vi "in_1d interp.vi"(7 "method":i32(ring) items=["nearest", "linear", "spline", "cubic Hermite", "Lagrange"], 9 "xi":dbl[](array[numeric]), 10 "Y":dbl[](array[numeric]), 11 "X":dbl[](array[numeric])) -> (0 "error":i32, 3 "yi":dbl[](array[numeric]))   [LabVIEW 2020, in "NI_Gmath.lvlib"]
uses:
  NI_Gmath.lvlib
  Scalar Polynomial Evaluation (DBL).vi
  NI_AALPro.lvlib
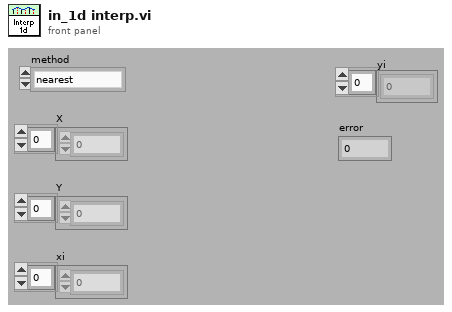
[diagram p1: front panel]
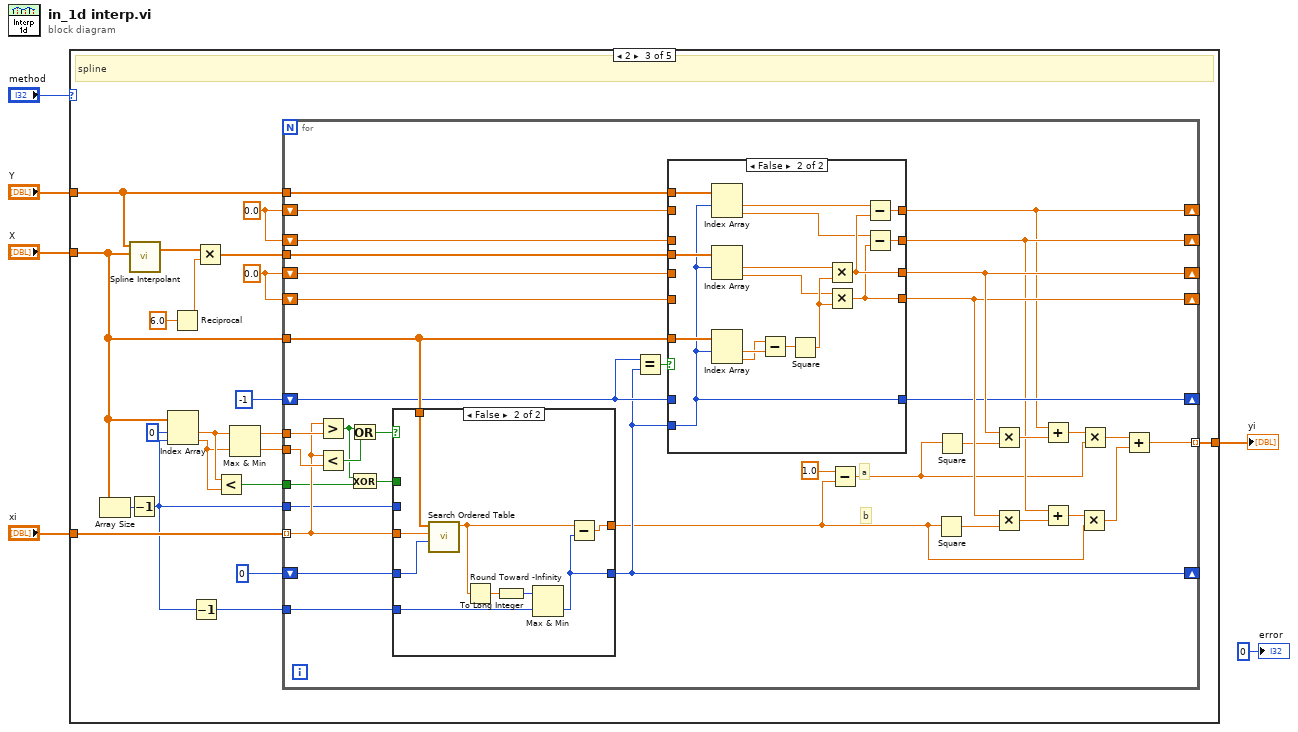
[diagram p0: block diagram]
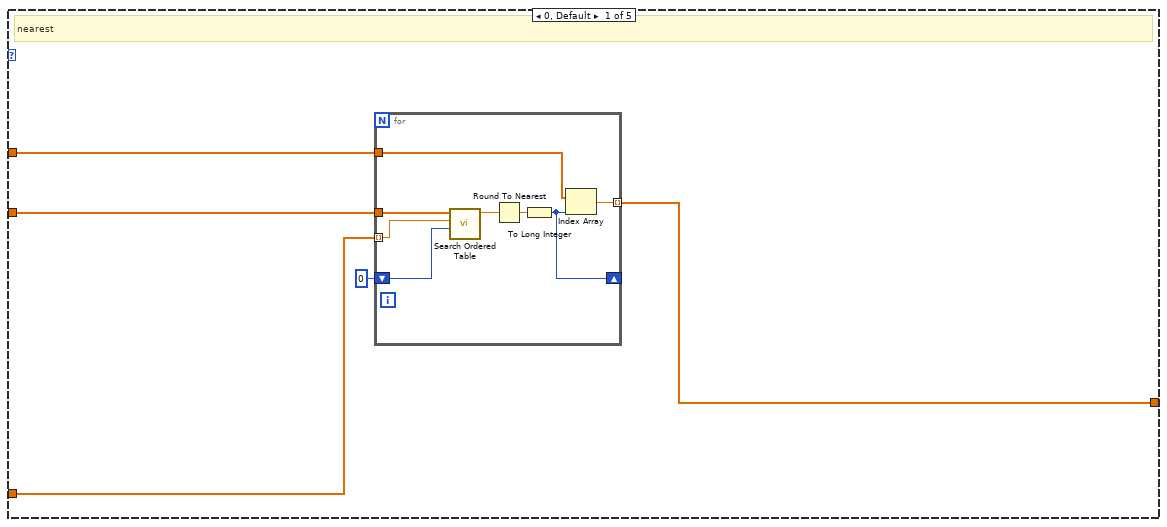
[diagram p2: hidden frame]
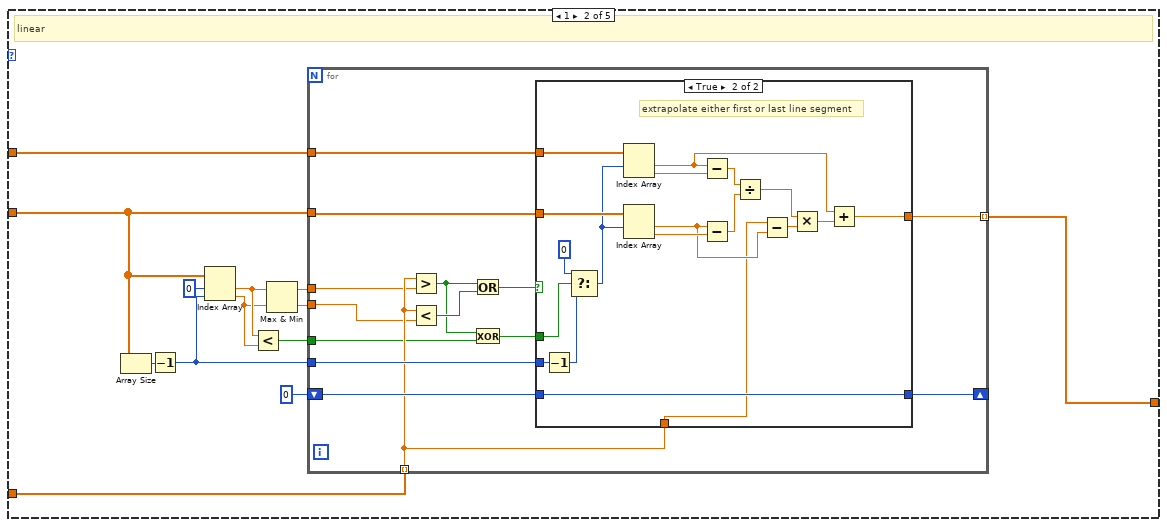
[diagram p3: hidden frame]
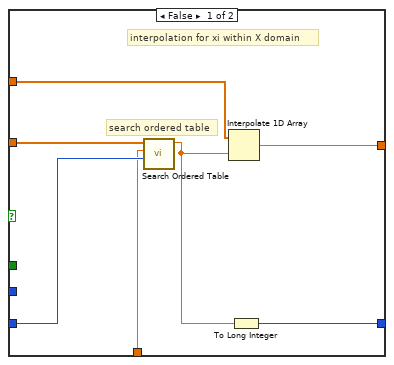
[diagram p4: hidden frame]
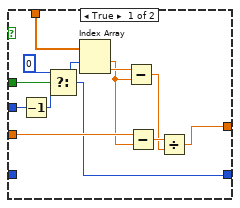
[diagram p5: hidden frame]
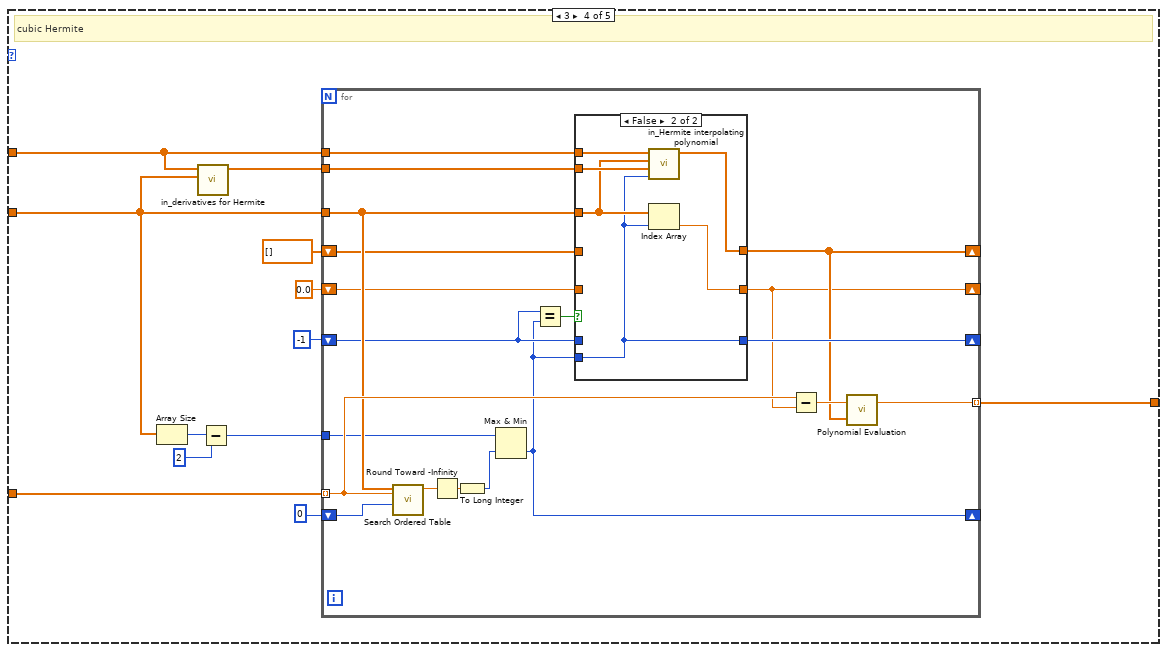
[diagram p7: hidden frame]
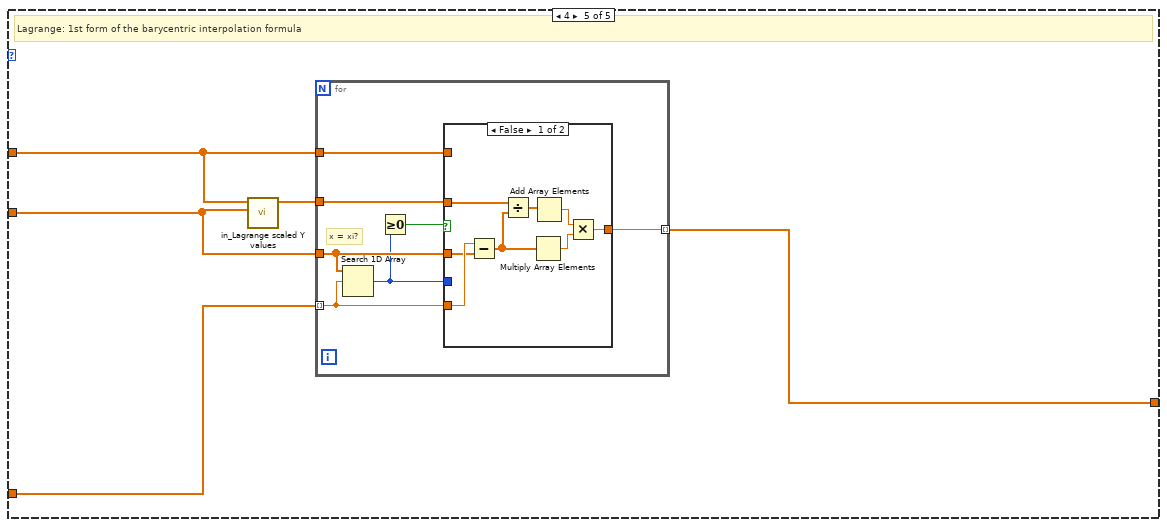
[diagram p9: hidden frame]
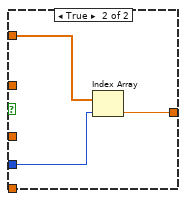
[diagram p10: hidden frame]
diagram:
  n1 = case shown="2" "method" {
    tunnel: "Y" -> [w7 w32 w93 w182 w214]
    tunnel: "X" -> [w9 w29 w78 w175 w217]
    tunnel: "xi" -> [w11 w26 w90 w185 w218]
    tunnel: [w10 w25 w92 w183 w215] -> w3
    frame 0, Default {
      # "nearest"
      n2 = for {
        tunnel: w9 -> [w16]
        tunnel: w11 -> [w15] mode=indexing
        tunnel: w7 -> [w18]
        tunnel: [w17] -> w10 mode=indexing
        shift-right: [w12] -> _
        shift-left: 0 -> [w14]
        n3 = call "Search Ordered Table.vi"("starting index"=w14, "x value"=w15, "ordered x array"=w16) -> ("fractional index"=w13:dbl)  [unwired: 8 in]
        n4 = Round To Nearest(number=w13) -> (nearest integer value=w19:dbl)
        n5 = To Long Integer(number=w19) -> (32bit integer=w12:i32)
        n6 = Index Array(array=w18, index=w12) -> (element=w17:dbl)
      }
    }
    frame 1 {
      # "linear"
      n7 = Array Size(array=w29) -> (size(s)=w30:i32)
      n8 = Decrement(x=w30) -> (x-1=w28:i32)
      n9 = Index Array(array=w29, index #1=0 ("index"), index #2=w28) -> (element #1=w23:dbl, element #2=w22:dbl)
      n10 = Less?(x=w23, y=w22) -> (x < y?=w24:bool)
      n11 = Max & Min(x=w23, y=w22) -> (max(x,y)=w21:dbl, min(x,y)=w20:dbl)
      n12 = for {
        tunnel: w29 -> [w46]
        tunnel: w32 -> [w45]
        tunnel: [w44] -> w25 mode=indexing
        tunnel: w20 -> [w33]
        tunnel: w21 -> [w34]
        tunnel: w28 -> [w42]
        shift-right: [w40] -> _
        shift-left: 0 ("index") -> [w41]
        tunnel: w26 -> [w39] mode=indexing
        tunnel: w24 -> [w38]
        n13 = Greater?(x=w39, y=w34) -> (0:w35:bool)
        n14 = Less?(x=w39, y=w33) -> (x < y?=w37:bool)
        n15 = Or(x=w35, y=w37) -> (x .or. y?=w43:bool)
        n16 = Exclusive Or(1:w38, 2:w35) -> (0:w36:bool)
        n17 = case shown="True" w43 {
          tunnel: w46 -> [w51 w72]
          tunnel: w45 -> [w53 w71]
          tunnel: [w52 w70] -> w44
          tunnel: w36 -> [_ w58]
          tunnel: w42 -> [_ w69]
          tunnel: w41 -> [w50 w55]
          tunnel: [w47 w55] -> w40
          tunnel: w39 -> [w49 w54]
          frame False {
            # "search ordered table"
            # "interpolation for xi within X domain"
            n18 = call "Search Ordered Table.vi"("starting index"=w50, "x value"=w49, "ordered x array"=w51) -> ("fractional index"=w48:dbl)  [unwired: 8 in]
            n19 = Interpolate 1D Array(1:w48, 2:w53) -> (0:w52:dbl)
            n20 = To Long Integer(number=w48) -> (32bit integer=w47:i32)
          }
          frame True {
            # "extrapolate either first or last line segment"
            n21 = Decrement(x=w69) -> (x-1=w59:i32)
            n22 = Select(t=0, s=w58, f=w59) -> (s? t:f=w56:i32)
            n23 = Index Array(array=w71, index #1=w56) -> (element #1=w66:dbl, element #2=w68:dbl)  [unwired: 1 in]
            n24 = Index Array(array=w72, index #1=w56) -> (element #1=w65:dbl, element #2=w67:dbl)  [unwired: 1 in]
            n25 = Subtract(x=w66, y=w68) -> (x-y=w64:dbl)
            n26 = Subtract(x=w65, y=w67) -> (x-y=w63:dbl)
            n27 = Divide(x=w64, y=w63) -> (x/y=w61:dbl)
            n28 = Subtract(x=w54, y=w65) -> (x-y=w62:dbl)
            n29 = Multiply(x=w61, y=w62) -> (x*y=w60:dbl)
            n30 = Add(x=w66, y=w60) -> (x+y=w70:dbl)
          }
        }
      }
    }
    frame 2 {
      w83 = 0.0
      w84 = 0.0 ("Numeric")
      # "spline"
      n31 = Array Size(array=w78) -> (size(s)=w81:i32)
      n32 = Decrement(x=w81) -> (x-1=w74:i32)
      n33 = call "Spline Interpolant.vi"("X"=w78, "Y"=w93) -> ("Interpolant"=w87:dbl[])  [unwired: 2 in, 1 out]
      n34 = Index Array(array=w78, index #1=0 ("index"), index #2=w74) -> (element #1=w80:dbl, element #2=w79:dbl)
      n35 = Reciprocal(x=6.0) -> (1/x=w88:dbl)
      n36 = Decrement(x=w74) -> (x-1=w73:i32)
      n37 = Multiply(x=w87, y=w88) -> (x*y=w86:dbl[])
      n38 = Less?(x=w80, y=w79) -> (x < y?=w77:bool)
      n39 = Max & Min(x=w80, y=w79) -> (max(x,y)=w76:dbl, min(x,y)=w75:dbl)
      n40 = for {
        tunnel: w93 -> [w130]
        tunnel: w78 -> [w129]
        tunnel: [w126] -> w92 mode=indexing
        shift-right: [w96] -> _
        shift-left: 0 -> [w131]
        tunnel: w90 -> [w101] mode=indexing
        tunnel: w86 -> [w128]
        shift-right: [w117] -> _
        shift-left: -1 -> [w118]
        shift-right: [w112] -> _
        shift-left: w84 -> [w124]
        shift-right: [w114] -> _
        shift-left: w84 -> [w123]
        shift-right: [w122] -> _
        shift-left: w83 -> [w120]
        shift-right: [w121] -> _
        shift-left: w83 -> [w119]
        tunnel: w74 -> [w98]
        tunnel: w77 -> [w100]
        tunnel: w76 -> [w103]
        tunnel: w75 -> [w102]
        tunnel: w73 -> [w94]
        # "a"
        # "b"
        n41 = Greater?(x=w101, y=w103) -> (0:w104:bool)
        n42 = Less?(x=w101, y=w102) -> (x < y?=w105:bool)
        n43 = Or(x=w104, y=w105) -> (x .or. y?=w99:bool)
        n44 = Exclusive Or(1:w100, 2:w104) -> (0:w97:bool)
        n45 = case shown="False" w99 {
          tunnel: w131 -> [_ w152]
          tunnel: w129 -> [w138 w151]
          tunnel: [w133 w147] -> w95
          tunnel: w101 -> [w137 w150]
          tunnel: w98 -> [w141 _]
          tunnel: w97 -> [w140 _]
          tunnel: [w132 w144] -> w96
          tunnel: w94 -> [_ w146]
          frame True {
            n46 = Decrement(x=w141) -> (x-1=w143:i32)
            n47 = Select(t=0, s=w140, f=w143) -> (s? t:f=w132:i32)
            n48 = Index Array(array=w138, index #1=w132) -> (element #1=w136:dbl, element #2=w139:dbl)  [unwired: 1 in]
            n49 = Subtract(x=w139, y=w136) -> (x-y=w134:dbl)
            n50 = Subtract(x=w137, y=w136) -> (x-y=w135:dbl)
            n51 = Divide(x=w135, y=w134) -> (x/y=w133:dbl)
          }
          frame False {
            n52 = call "Search Ordered Table.vi"("starting index"=w152, "x value"=w150, "ordered x array"=w151) -> ("fractional index"=w148:dbl)  [unwired: 8 in]
            n53 = Round Toward -Infinity(1:w148) -> (0:w149:dbl)
            n54 = To Long Integer(number=w149) -> (32bit integer=w145:i32)
            n55 = Max & Min(x=w145, y=w146) -> (min(x,y)=w144:i32)  [unwired: 1 out]
            n56 = Subtract(x=w148, y=w144) -> (x-y=w147:dbl)
          }
        }
        n57 = Equal?(x=w118, y=w96) -> (x = y?=w125:bool)
        n58 = case shown="False" w125 {
          tunnel: w130 -> [_ w173]
          tunnel: w129 -> [_ w172]
          tunnel: w128 -> [_ w171]
          tunnel: [w155 w162] -> w122
          tunnel: [w154 w159] -> w121
          tunnel: [w157 w161] -> w112
          tunnel: [w156 w158] -> w114
          tunnel: w96 -> [_ w164]
          tunnel: w124 -> [w157 _]
          tunnel: w123 -> [w156 _]
          tunnel: w120 -> [w155 _]
          tunnel: w119 -> [w154 _]
          tunnel: w118 -> [w153 _]
          tunnel: [w153 w164] -> w117
          frame True {
          }
          frame False {
            n59 = Index Array(array=w173, index #1=w164) -> (element #1=w163:dbl, element #2=w160:dbl)  [unwired: 1 in]
            n60 = Index Array(array=w171, index #1=w164) -> (element #1=w166:dbl, element #2=w165:dbl)  [unwired: 1 in]
            n61 = Index Array(array=w172, index #1=w164) -> (element #1=w168:dbl, element #2=w167:dbl)  [unwired: 1 in]
            n62 = Subtract(x=w167, y=w168) -> (x-y=w170:dbl)
            n63 = Square(x=w170) -> (x^2=w169:dbl)
            n64 = Multiply(x=w166, y=w169) -> (x*y=w162:dbl)
            n65 = Multiply(x=w165, y=w169) -> (x*y=w159:dbl)
            n66 = Subtract(x=w163, y=w162) -> (x-y=w161:dbl)
            n67 = Subtract(x=w160, y=w159) -> (x-y=w158:dbl)
          }
        }
        n68 = Subtract(x=1.0, y=w95) -> (x-y=w109:dbl)
        n69 = Square(x=w95) -> (x^2=w107:dbl)
        n70 = Square(x=w109) -> (x^2=w115:dbl)
        n71 = Multiply(x=w122, y=w115) -> (x*y=w116:dbl)
        n72 = Multiply(x=w121, y=w107) -> (x*y=w108:dbl)
        n73 = Add(x=w112, y=w116) -> (x+y=w111:dbl)
        n74 = Add(x=w114, y=w108) -> (x+y=w106:dbl)
        n75 = Multiply(x=w106, y=w95) -> (x*y=w113:dbl)
        n76 = Multiply(x=w111, y=w109) -> (x*y=w110:dbl)
        n77 = Add(x=w110, y=w113) -> (x+y=w126:dbl)
      }
    }
    frame 3 {
      # "cubic Hermite"
      n78 = Array Size(array=w175) -> (size(s)=w177:i32)
      n79 = call "in_derivatives for Hermite.vi"("Y[0..N]"=w182, "X[0..N]"=w175) -> ("Y deriv[0..N]"=w184:dbl[])  [unwired: 8 in]
      n80 = Subtract(x=w177, y=2) -> (x-y=w174:i32)
      n81 = for {
        tunnel: w175 -> [w196]
        tunnel: w185 -> [w198] mode=indexing
        tunnel: w182 -> [w204]
        tunnel: w184 -> [w201]
        tunnel: [w202] -> w183 mode=indexing
        shift-right: [w186] -> _
        shift-left: 0 -> [w197]
        shift-right: [w193] -> _
        shift-left: -1 -> [w195]
        shift-right: [w192] -> _
        shift-left: dbl[] [] ("Hermite polynomial") -> [w190]
        shift-right: [w191] -> _
        shift-left: 0.0 ("Numeric") -> [w189]
        tunnel: w174 -> [w188]
        n82 = call "Search Ordered Table.vi"("starting index"=w197, "x value"=w198, "ordered x array"=w196) -> ("fractional index"=w203:dbl)  [unwired: 8 in]
        n83 = Round Toward -Infinity(1:w203) -> (0:w200:dbl)
        n84 = To Long Integer(number=w200) -> (32bit integer=w187:i32)
        n85 = Max & Min(x=w188, y=w187) -> (min(x,y)=w186:i32)  [unwired: 1 out]
        n86 = Equal?(x=w195, y=w186) -> (x = y?=w194:bool)
        n87 = case shown="False" w194 {
          tunnel: w204 -> [_ w213]
          tunnel: [w206 w212] -> w192
          tunnel: w201 -> [_ w211]
          tunnel: [w205 w210] -> w191
          tunnel: w186 -> [_ w208]
          tunnel: w196 -> [_ w209]
          tunnel: w195 -> [w207 _]
          tunnel: [w207 w208] -> w193
          tunnel: w190 -> [w206 _]
          tunnel: w189 -> [w205 _]
          frame True {
          }
          frame False {
            n88 = call "in_Hermite interpolating polynomial.vi"("index i"=w208, "Y deriv[0..N]"=w211, "X[0..N]"=w209, "Y[0..N]"=w213) -> ("Hermite polynomial"=w212:dbl[])  [unwired: 7 in]
            n89 = Index Array(array=w209, index=w208) -> (element=w210:dbl)
          }
        }
        n90 = Subtract(x=w198, y=w191) -> (x-y=w199:dbl)
        n91 = call-poly "Polynomial Evaluation.vi"("P(x)"=w192, "a"=w199) -> ("P(a)"=w202:dbl)  [unwired: 1 out]
      }
    }
    frame 4 {
      # "Lagrange: 1st form of the barycentric interpolation formula"
      n92 = call "in_Lagrange scaled Y values.vi"("X[0..N]"=w217, "Y[0..N]"=w214) -> ("scaled Y"=w216:dbl[])  [unwired: 9 in]
      n93 = for {
        tunnel: w217 -> [w221]
        tunnel: w218 -> [w220] mode=indexing
        tunnel: w216 -> [w225]
        tunnel: [w224] -> w215 mode=indexing
        tunnel: w214 -> [w222]
        # "x = xi?"
        n94 = Search 1D Array(1D array=w221, element=w220) -> (index of element=w219:i32)  [unwired: 1 in]
        n95 = Greater Or Equal To 0?(x=w219) -> (x >= 0?=w223:bool)
        n96 = case shown="False" w223 {
          tunnel: w220 -> [w233 _]
          tunnel: w221 -> [w232 _]
          tunnel: w225 -> [w231 _]
          tunnel: [w227 w234] -> w224
          tunnel: w222 -> [_ w236]
          tunnel: w219 -> [_ w235]
          frame False {
            n97 = Subtract(x=w233, y=w232) -> (x-y=w226:dbl[])
            n98 = Divide(x=w231, y=w226) -> (x/y=w229:dbl[])
            n99 = Multiply Array Elements(1:w226) -> (0:w230:dbl)
            n100 = Add Array Elements(numeric array=w229) -> (sum=w228:dbl)
            n101 = Multiply(x=w228, y=w230) -> (x*y=w227:dbl)
          }
          frame True {
            n102 = Index Array(array=w236, index=w235) -> (element=w234:dbl)
          }
        }
      }
    }
  }
  "yi" <- w3
  "error" <- 0 ("error")
